vi "一体站流程平行样自动启动.vi"(11 "参数":T1) -> ()   [LabVIEW 2016, in "质控单元.lvlib"]
panel:
  out "枚举":enum16{"初始化", "采配水启动", "等待", "配水", "排水", "结束"}(ring)
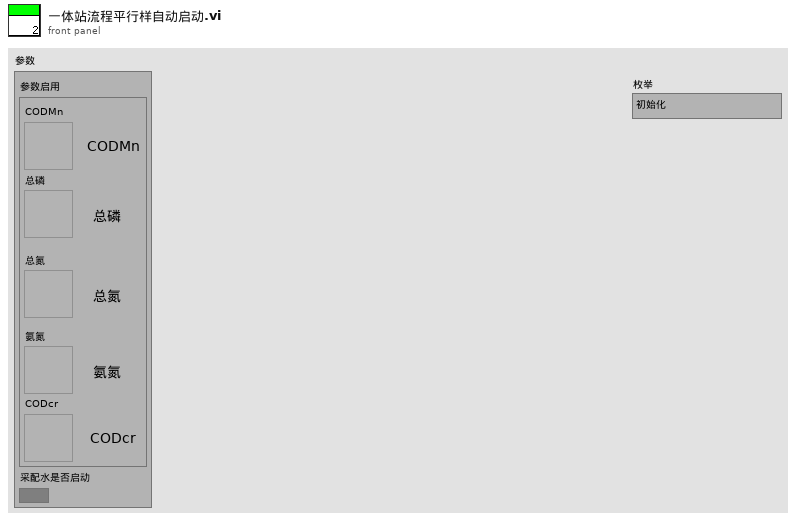
[diagram p1: front panel]
types:
  T1 = cluster{"参数启用":cluster{"CODMn":bool, "总磷":bool, "总氮":bool, "氨氮":bool, "CODcr":bool}, "采配水是否启动":bool}
  T2 = cluster{"命令":string, cluster{"starting address":u16, "holding register value":u16}}
  T3 = typedef "质控单元.lvlib/平行样测试流程.ctl" = enum16{"待机", "第一次水样测试启动", "第一次水样测试中", "第二次水样测试启动", "第二次水样测试中", "存储平行样测试数据", "结束"}
  T4 = cluster{"站号":u16, "量程切换":enum32{"H", "L", "AUTO"}, "控制命令":enum16{"启动测量", "标样核查", "零点核查", "跨度核查", "空白测试", "平行样测试", "加标回收", "空白校准", "标样校准", "初始化（清洗）", "停止测试", "仪器重启", "校时", "模式设置", "测量间隔设置"}, "模式设置":enum16{"待机", "连续模式", "周期模式", "定点模式", "受控模式", "手动模式"}, "测量间隔":u16}
  T5 = cluster{"时间标识":timestamp, "设备":string, "日志信息":string}
  T6 = enum16{"空闲", "水样测试", "标样核查", "零点核查", "跨度核查", "空白测试", "平行样测试", "加标回收", "空白校准", "标样校准", "初始化（清洗）"}
  T7 = cluster{"测量模式":enum16{"水样测量", "标样核查", "零点核查", "跨度核查", "空白测试", "加标回收", "平行样", "校零", "校标"}}
  T8 = cluster{"时间标识":timestamp, "设备":string, "日志信息":string, "流程参数":string}
  T9 = cluster{"R0":i16, "R1":i16, "R2":i16, "R3":i16, "R4":i16, "R5":i16, "R6":i16, "R7":i16, "R8":i16, "R9":i16, "R10":i16, "R11":i16, "R12":i16, "R13":i16, "R14":i16, "R15":i16, "R16":i16, "R17":i16, "R18":i16, "R19":i16, "R20":i16, "R21":i16, "R22":i16, "R23":i16, "R24":i16, "R25":i16, "R26":i16, "R27":i16, "R28":i16, "R29":i16, "R30":i16, "R31":i16, "R32":i16, "R33":i16, "R34":i16, "R35":i16, "R36":i16, "R37":i16, "R38":i16, "R39":i16, "R40":i16, "R41":i16, "R42":i16, "R43":i16, "R44":i16, "R45":i16, "R46":i16, "R47":i16, "R48":i16, "R49":i16, "R50":i16, "R51":i16, "R52":i16, "R53":i16, "R54":i16, "R55":i16, "R56":i16}
  T10 = cluster{"系统时间":timestamp, "工作状态":enum16{"空闲", "水样测试", "标样核查", "零点核查", "跨度核查", "空白测试", "平行样测试", "加标回收", "空白校准", "标样校准", "初始化（清洗）"}, "测量模式":enum16{"待机", "连续模式", "周期模式", "定点模式", "受控模式", "手动模式"}, "告警代码":enum16{"无告警", "缺试剂告警", "缺水样告警", "缺蒸馏水告警", "缺标液告警", "仪表漏液告警", "标定异常告警", "超量程告警", "加热异常", "低试剂预警", "超上限告警", "超下限告警", "仪表内部其他异常", "滴定异常告警", "电极异常告警", "量程切换告警", "参数设置告警", "PH电极电位异常", "电导率电极异常", "浊度光度异常", "溶解氧电极异常", "溶解氧光强异常", "温度异常告警", "PH异常告警", "溶解氧异常告警", "电导率异常告警", "浊度异常告警", "叶绿素异常告警", "藻密度异常告警", "蓝绿藻异常告警", "ORP异常告警", "氨氮异常告警", "清洁刷异常告警", "SD卡异常告警", "蓝牙异常告警", "Wifi异常告警", "流程异常告警"}, "故障代码":enum16{"无故障", "电机故障", "温度故障", "通讯故障", "滴定故障"}, "日志代码":u16, "软件版本":u16, "F0":sgl, "F1":sgl, "F2":sgl, "F3":sgl, "T":sgl, "H":sgl, "id":u16, "flowid":u16, "量程":u16, "总磷控温温度1":sgl, "营养盐控温温度2":sgl, "ADC":sgl}
  T11 = cluster{"因子编码":u32, "单位":u16, "标样参考值":sgl, "水样数据时间":timestamp, "水样实测值":sgl, "水样数据标识":string, "标样数据时间":timestamp, "标样实测值":sgl, "标样数据标识":string, "空白数据时间":timestamp, "空白实测值":sgl, "空白数据标识":string, "零点核查数据时间":timestamp, "零点核查实测值":sgl, "零点核查数据标识":string, "跨度核查数据时间":timestamp, "跨度核查实测值":sgl, "跨度核查数据标识":string, "加标回收数据时间":timestamp, "加标回收实测值":sgl, "加标回收数据标识":string, "平行样数据时间":timestamp, "平行样实测值":sgl, "平行样数据标识":string}
  T12 = cluster{"时间标识":timestamp, "参数":string, "第一次水样浓度值":sgl, "第二次水样测试时间":timestamp, "第二次水样浓度值":sgl}
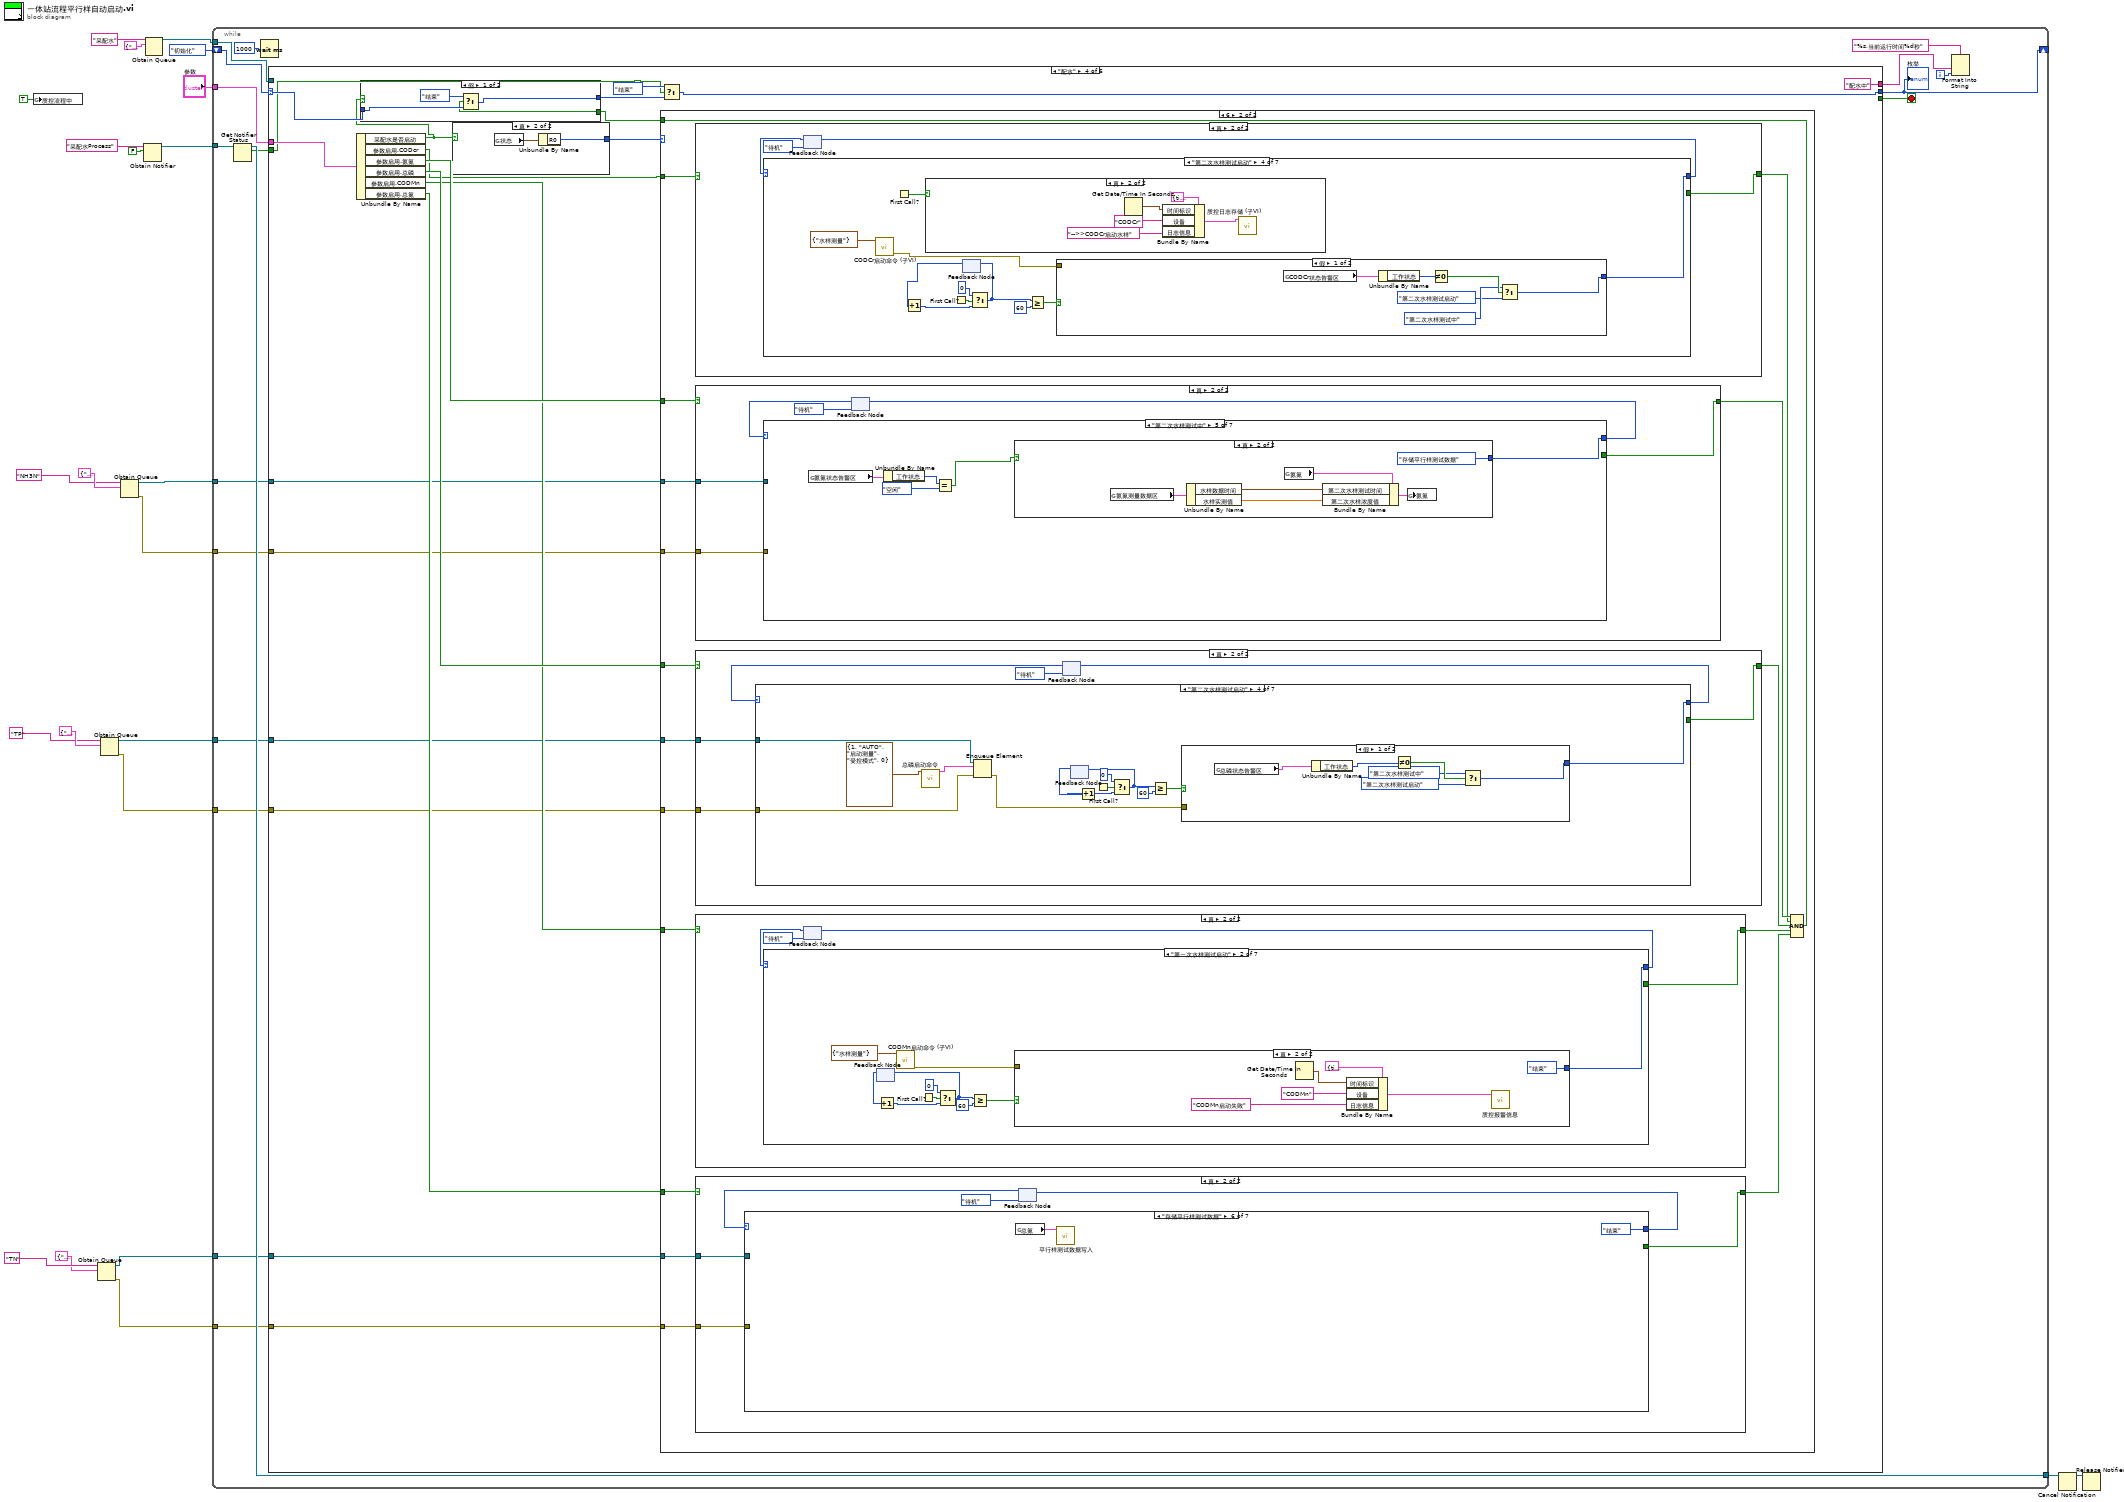
[diagram p0: block diagram]
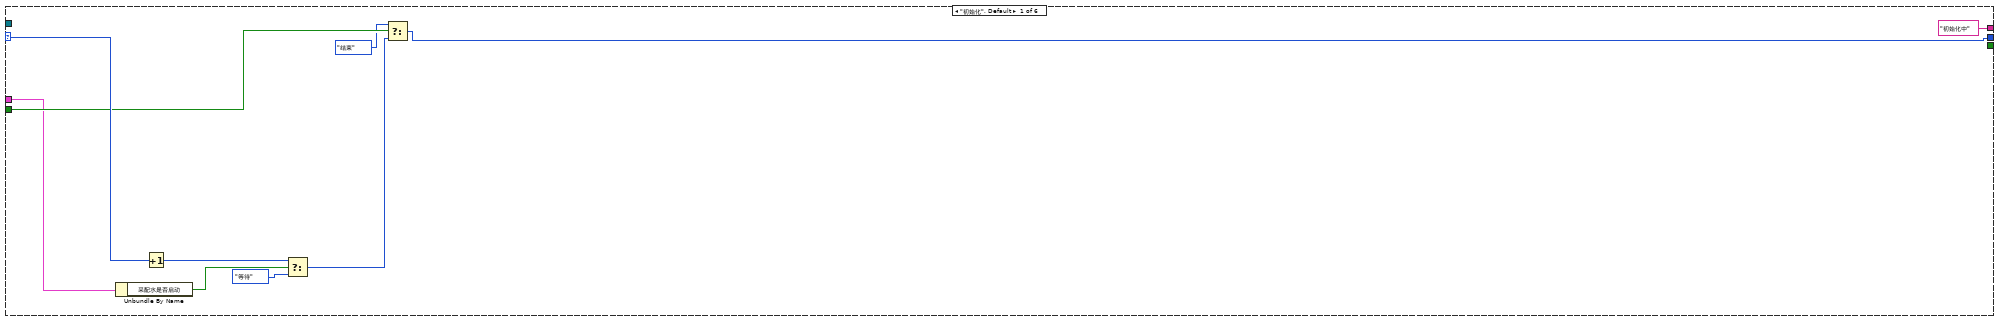
[diagram p2: hidden frame]
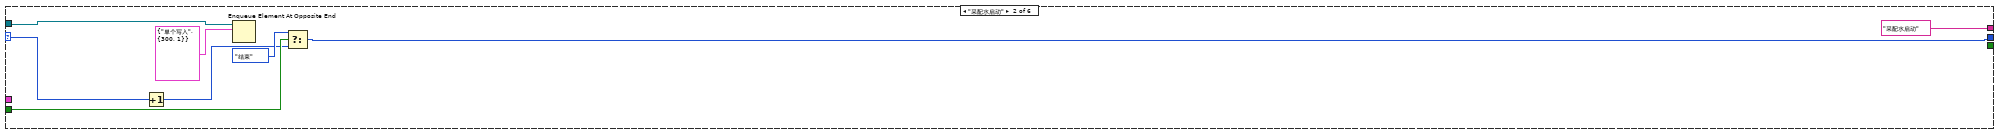
[diagram p3: hidden frame]
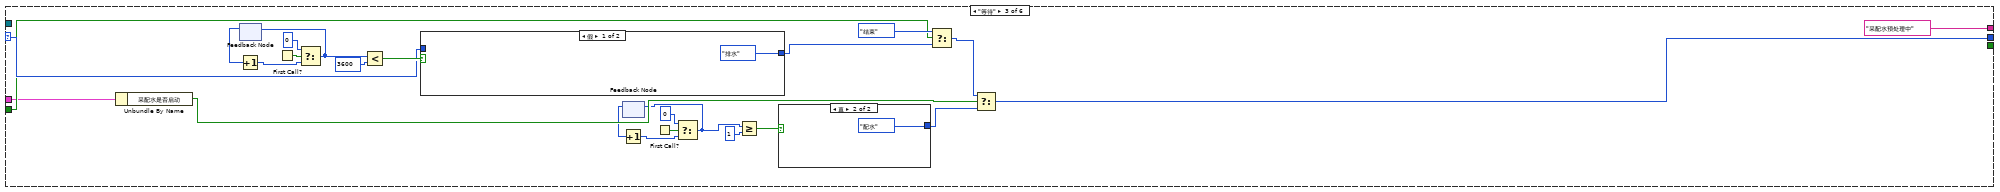
[diagram p4: hidden frame]
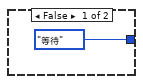
[diagram p5: hidden frame]
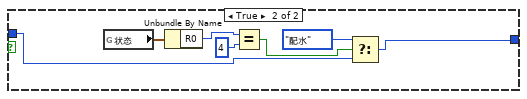
[diagram p6: hidden frame]
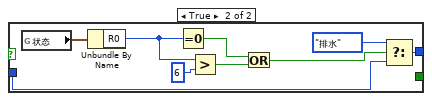
[diagram p7: hidden frame]
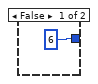
[diagram p8: hidden frame]
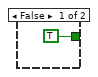
[diagram p10: hidden frame]
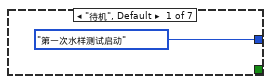
[diagram p11: hidden frame]
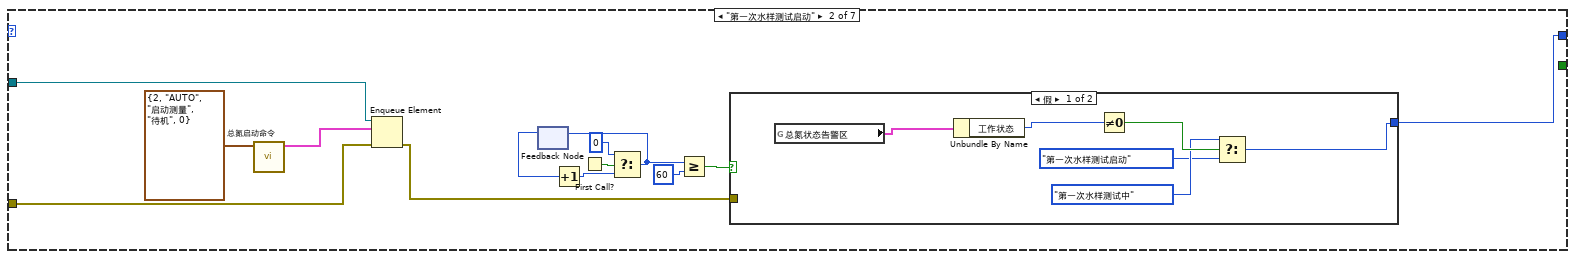
[diagram p12: hidden frame]
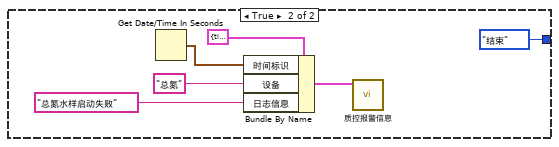
[diagram p13: hidden frame]
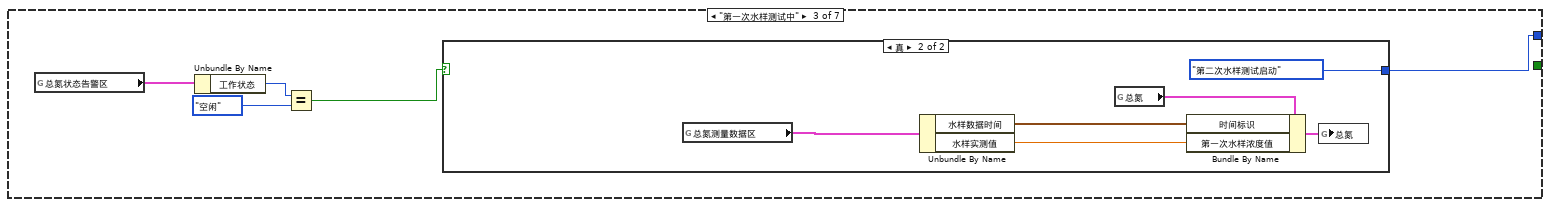
[diagram p14: hidden frame]
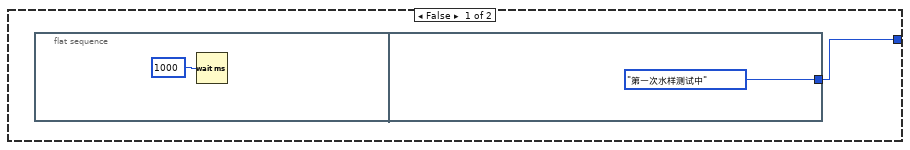
[diagram p15: hidden frame]
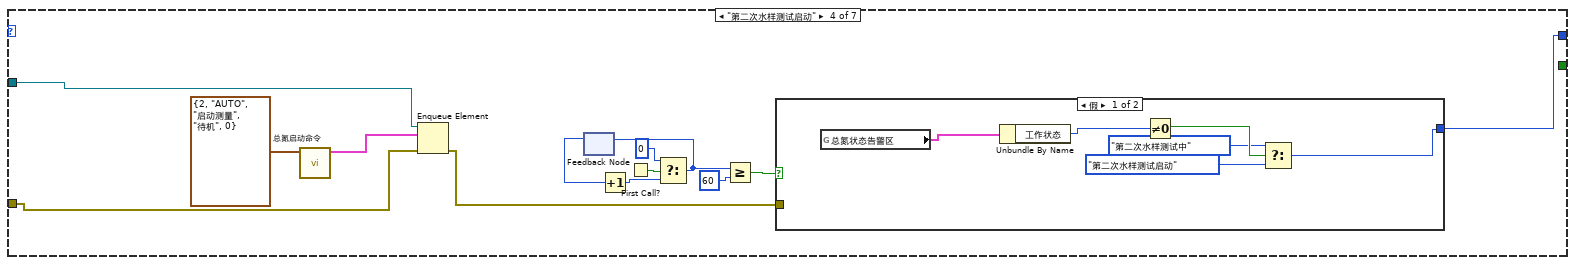
[diagram p16: hidden frame]
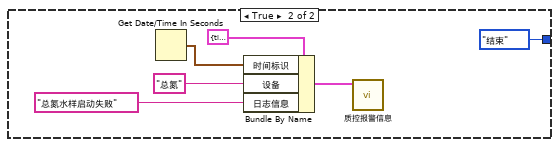
[diagram p17: hidden frame]
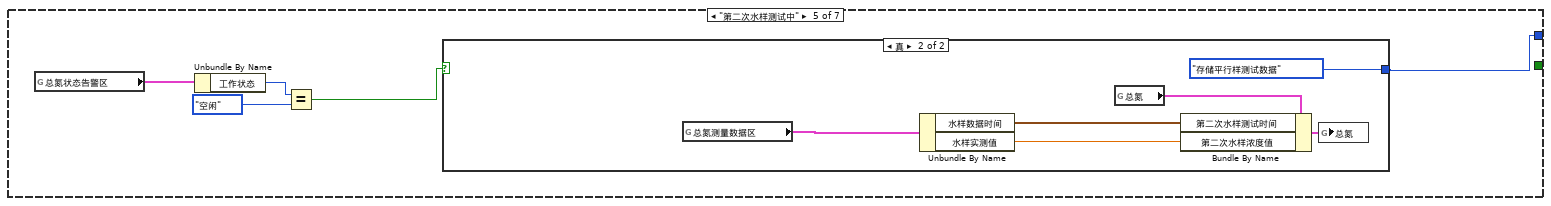
[diagram p18: hidden frame]
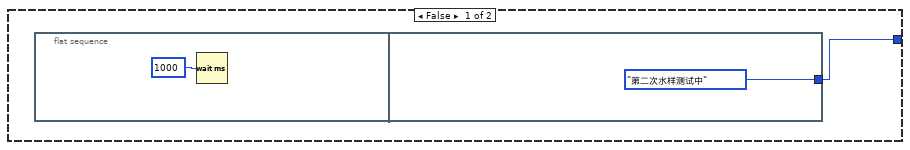
[diagram p19: hidden frame]
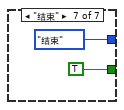
[diagram p20: hidden frame]
diagram:
  n1 = global write "质控测完标志全局 1.vi" "质控流程中"(TRUE ("质控流程中")) -> ()
  n2 = Obtain Queue(name (unnamed)="TN" ("名称（未命名）"), element data type=cluster{"命令":string, "data":variant} {"命令"="", "data"=variant}) -> (queue out=w3:refnum<queue>, error out=w2:errorcluster)  [unwired: 3 in, 1 out]
  n3 = Obtain Queue(name (unnamed)="TP" ("名称（未命名）"), element data type=cluster{"命令":string, "data":variant} {"命令"="", "data"=variant}) -> (queue out=w5:refnum<queue>, error out=w4:errorcluster)  [unwired: 3 in, 1 out]
  n4 = Obtain Queue(name (unnamed)="NH3N" ("名称（未命名）"), element data type=cluster{"命令":string, "data":variant} {"命令"="", "data"=variant}) -> (queue out=w7:refnum<queue>, error out=w6:errorcluster)  [unwired: 3 in, 1 out]
  n5 = Obtain Notifier(name (unnamed)="采配水Process" ("名称（未命名）"), notification data type=FALSE) -> (notifier out=w16:refnum<notifier>)  [unwired: 2 in, 2 out]
  n6 = Obtain Queue(name (unnamed)="采配水" ("名称（未命名）"), element data type=cluster{"命令":string, "数据":variant} {"命令"="", "数据"=variant}) -> (queue out=w21:refnum<queue>)  [unwired: 3 in, 2 out]
  n7 = while {
    tunnel: w21 -> [w41]
    shift-right: [w39] -> _
    shift-left: enum16{"初始化", "采配水启动", "等待", "配水", "排水", "结束"}."初始化" ("枚举") -> [w40]
    tunnel: "参数" -> [w37]
    tunnel: w16 -> [w36]
    tunnel: [w35] -> w15
    tunnel: w7 -> [w30]
    tunnel: w6 -> [w29]
    tunnel: w5 -> [w28]
    tunnel: w4 -> [w27]
    tunnel: w3 -> [w26]
    tunnel: w2 -> [w25]
    i -> [w32]
    stop <- w24 stop-if-true
    n8 = Get Notifier Status(notifier=w36) -> (notifier out=w35:refnum<notifier>, current notification=w31:bool)  [unwired: 1 in, 3 out]
    n9 = Wait (ms)(milliseconds to wait=u32 1000 ("等待时间（毫秒）")) -> ()  [unwired: 1 out]
    n10 = case shown="\"配水\"" w40 {
      selector: w40 -> [w51 w57 w81 w114 w591 w598]
      tunnel: w41 -> [_ w58 _ _ w592 _]
      tunnel: [w48 w52 w60 w111 w586 w597] -> w39
      tunnel: [_ _ _ _ _ TRUE] -> w24
      tunnel: w37 -> [w46 _ w71 w107 _ _]
      tunnel: ["初始化中" ("输入 1") "采配水启动" ("输入 1") "采配水预处理中" ("输入 1") "配水中" ("输入 1") "排水中" ("输入 1") "结束" ("输入 1")] -> w33
      tunnel: w31 -> [w49 w54 w73 w95 w588 _]
      tunnel: w30 -> [_ _ _ w102 _ _]
      tunnel: w29 -> [_ _ _ w101 _ _]
      tunnel: w28 -> [_ _ _ w100 _ _]
      tunnel: w27 -> [_ _ _ w99 _ _]
      tunnel: w26 -> [_ _ _ w98 _ _]
      tunnel: w25 -> [_ _ _ w97 _ _]
      frame "初始化", Default {
        n11 = Unbundle By Name(w46) -> ("采配水是否启动"=w45:bool)
        n12 = Increment(x=w51) -> (x+1=w44:enum16{"初始化", "采配水启动", "等待", "配水", "排水", "结束"})
        n13 = Select(t=w44, s=w45, f=enum16{"初始化", "采配水启动", "等待", "配水", "排水", "结束"}."等待") -> (s? t:f=w43:enum16{"初始化", "采配水启动", "等待", "配水", "排水", "结束"})
        n14 = Select(t=enum16{"初始化", "采配水启动", "等待", "配水", "排水", "结束"}."结束", s=w49, f=w43) -> (s? t:f=w48:enum16{"初始化", "采配水启动", "等待", "配水", "排水", "结束"})
      }
      frame "采配水启动" {
        n15 = Increment(x=w57) -> (x+1=w53:enum16{"初始化", "采配水启动", "等待", "配水", "排水", "结束"})
        n16 = Enqueue Element At Opposite End(queue=w58, element=T2 {"命令"="单个写入", {"starting address"=300, "holding register value"=1}} ("元素")) -> ()  [unwired: 2 in, 3 out]
        n17 = Select(t=enum16{"初始化", "采配水启动", "等待", "配水", "排水", "结束"}."结束", s=w54, f=w53) -> (s? t:f=w52:enum16{"初始化", "采配水启动", "等待", "配水", "排水", "结束"})
      }
      frame "等待" {
        n18 = Unbundle By Name(w71) -> ("采配水是否启动"=w70:bool)
        n19 = feedback #1() -> (w78:i32)  [unwired: 1 in]
        n20 = Increment(x=w78) -> (x+1=w77:i32)
        n21 = First Call?() -> (First Call?: T/F=w79:bool)
        n22 = Select(t=0, s=w79, f=w77) -> (s? t:f=w76:i32)
        n23 = feedback-in #1(w76) -> ()
        n24 = Less?(x=w76, y=3600) -> (x < y?=w82:bool)
        n25 = case shown="假" w82 {
          tunnel: w81 -> [_ w88]
          tunnel: [enum16{"初始化", "采配水启动", "等待", "配水", "排水", "结束"}."排水" ("枚举") w87] -> w72
          frame False {
          }
          frame True {
            n26 = global read "与采配水交互全局.vi" "状态"() -> (w93:T9)
            n27 = Unbundle By Name(w93) -> ("R0"=w92:i16)
            n28 = Equal?(x=w92, y=i16 4) -> (x = y?=w90:bool)
            n29 = Select(t=enum16{"初始化", "采配水启动", "等待", "配水", "排水", "结束"}."配水" ("枚举"), s=w90, f=w88) -> (s? t:f=w87:enum16{"初始化", "采配水启动", "等待", "配水", "排水", "结束"})
          }
        }
        n30 = feedback #2() -> (w66:i32)  [unwired: 1 in]
        n31 = Increment(x=w66) -> (x+1=w67:i32)
        n32 = First Call?() -> (First Call?: T/F=w65:bool)
        n33 = Select(t=0, s=w65, f=w67) -> (s? t:f=w68:i32)
        n34 = feedback-in #2(w68) -> ()
        n35 = Greater Or Equal?(x=w68, y=1) -> (x >= y?=w62:bool)
        n36 = case shown="真" w62 {
          tunnel: [enum16{"初始化", "采配水启动", "等待", "配水", "排水", "结束"}."等待" ("t") enum16{"初始化", "采配水启动", "等待", "配水", "排水", "结束"}."配水" ("t")] -> w61
          frame False {
          }
          frame True {
          }
        }
        n37 = Select(t=enum16{"初始化", "采配水启动", "等待", "配水", "排水", "结束"}."结束", s=w73, f=w72) -> (s? t:f=w69:enum16{"初始化", "采配水启动", "等待", "配水", "排水", "结束"})
        n38 = Select(t=w69, s=w70, f=w61) -> (s? t:f=w60:enum16{"初始化", "采配水启动", "等待", "配水", "排水", "结束"})
      }
      frame "配水" {
        n39 = Unbundle By Name(w107) -> ("采配水是否启动"=w96:bool, "参数启用.CODcr"=w106:bool, "参数启用.氨氮"=w110:bool, "参数启用.总磷"=w109:bool, "参数启用.CODMn"=w108:bool, "参数启用.总氮"=w105:bool)
        n40 = case shown="真" w96 {
          tunnel: [i16 6 ("R0") w129] -> w104
          frame False {
          }
          frame True {
            n41 = global read "与采配水交互全局.vi" "状态"() -> (w130:T9)
            n42 = Unbundle By Name(w130) -> ("R0"=w129:i16)
          }
        }
        n43 = case shown="6" w104 {
          tunnel: w110 -> [_ w147]
          tunnel: w109 -> [_ w146]
          tunnel: w108 -> [_ w143]
          tunnel: w106 -> [_ w142]
          tunnel: w105 -> [_ w139]
          tunnel: w102 -> [_ w137]
          tunnel: w101 -> [_ w136]
          tunnel: w100 -> [_ w135]
          tunnel: w99 -> [_ w134]
          tunnel: w98 -> [_ w133]
          tunnel: w97 -> [_ w132]
          tunnel: [_ w131] -> w94
          frame 0, Default {
          }
          frame 6 {
            n44 = case shown="真" w142 {
              tunnel: [TRUE w314] -> w141
              frame False {
              }
              frame True {
                n45 = feedback #3(平行样测试流程."待机") -> (w316:T3)
                n46 = case shown="\"第二次水样测试启动\"" w316 {
                  tunnel: [平行样测试流程."第一次水样测试启动" w328 w350 w370 w392 平行样测试流程."结束" 平行样测试流程."结束"] -> w315
                  tunnel: [_ _ _ _ _ _ TRUE] -> w314
                  frame "待机", Default {
                  }
                  frame "第一次水样测试启动" {
                    n47 = call "CODCr启动命令 (子VI).vi"("启动测量模式"=T7 {"测量模式"=enum."水样测量"}) -> ("错误输出"=w318:errorcluster)  [unwired: 10 in]
                    n48 = First Call?() -> (First Call?: T/F=w320:bool)
                    n49 = case shown="真" w320 {
                      frame False {
                      }
                      frame True {
                        n50 = Get Date/Time In Seconds() -> (seconds since 1Jan1904=w331:timestamp)
                        n51 = Bundle By Name(cluster=T8 {"时间标识"=timestamp(0 s since 1904-01-01), "设备"="", "日志信息"="", "流程参数"=""} ("data in"), "时间标识"=w331, "设备"="CODCr", "日志信息"="-->>CODCr启动水样") -> (w332:T8)
                        n52 = call "质控日志存储 (子VI).vi"("data in"=w332) -> ()  [unwired: 11 in]
                      }
                    }
                    n53 = feedback #4() -> (w324:i32)  [unwired: 1 in]
                    n54 = Increment(x=w324) -> (x+1=w325:i32)
                    n55 = First Call?() -> (First Call?: T/F=w323:bool)
                    n56 = Select(t=0, s=w323, f=w325) -> (s? t:f=w326:i32)
                    n57 = feedback-in #4(w326) -> ()
                    n58 = Greater Or Equal?(x=w326, y=60) -> (x >= y?=w321:bool)
                    n59 = case shown="假" w321 {
                      tunnel: [w338 平行样测试流程."结束"] -> w328
                      tunnel: w318 -> [_ _]
                      frame False {
                        n60 = global read "与CODCr交互全局.vi" "CODCr状态告警区"() -> (w335:T10)
                        n61 = Unbundle By Name(w335) -> ("工作状态"=w334:T6)
                        n62 = Not Equal To 0?(x=w334) -> (x != 0?=w339:bool)
                        n63 = Select(t=平行样测试流程."第一次水样测试中", s=w339, f=平行样测试流程."第一次水样测试启动") -> (s? t:f=w338:T3)
                      }
                      frame True {
                        n64 = Get Date/Time In Seconds() -> (seconds since 1Jan1904=w342:timestamp)
                        n65 = Bundle By Name(cluster=T5 {"时间标识"=timestamp(0 s since 1904-01-01), "设备"="", "日志信息"=""} ("data in"), "时间标识"=w342, "设备"="CODCr", "日志信息"="CODCr水样启动失败") -> (w340:T5)
                        n66 = call "质控报警信息.vi"("data in"=w340) -> ()  [unwired: 11 in]
                      }
                    }
                  }
                  frame "第一次水样测试中" {
                    n67 = global read "与CODCr交互全局.vi" "CODCr状态告警区"() -> (w349:T10)
                    n68 = Unbundle By Name(w349) -> ("工作状态"=w346:T6)
                    n69 = Equal?(x=w346, y=T6."空闲" ("工作状态")) -> (x = y?=w348:bool)
                    n70 = case shown="真" w348 {
                      tunnel: [w351 平行样测试流程."第二次水样测试启动"] -> w350
                      frame False {
                        n71 = flat-sequence {
                          tunnel: [平行样测试流程."第一次水样测试中"] -> w351
                          frame #0 {
                            n72 = Wait (ms)(milliseconds to wait=u32 1000 ("等待时间（毫秒）")) -> ()  [unwired: 1 out]
                          }
                          frame #1 {
                          }
                        }
                      }
                      frame True {
                        n73 = global read "与CODCr交互全局.vi" "CODCr测量数据区"() -> (w356:T11)
                        n74 = Unbundle By Name(w356) -> ("水样数据时间"=w355:timestamp, "水样实测值"=w354:sgl)
                        n75 = global read "平行样测试全局变量.vi" "CODcr"() -> (w358:T12)
                        n76 = Bundle By Name(cluster=w358, "时间标识"=w355, "第一次水样浓度值"=w354) -> (w357:T12)
                        n77 = global write "平行样测试全局变量.vi" "CODcr"(w357) -> ()
                      }
                    }
                  }
                  frame "第二次水样测试启动" {
                    n78 = call "CODCr启动命令 (子VI).vi"("启动测量模式"=T7 {"测量模式"=enum."水样测量"}) -> ("错误输出"=w360:errorcluster)  [unwired: 10 in]
                    n79 = First Call?() -> (First Call?: T/F=w362:bool)
                    n80 = case shown="真" w362 {
                      frame False {
                      }
                      frame True {
                        n81 = Get Date/Time In Seconds() -> (seconds since 1Jan1904=w373:timestamp)
                        n82 = Bundle By Name(cluster=T8 {"时间标识"=timestamp(0 s since 1904-01-01), "设备"="", "日志信息"="", "流程参数"=""} ("data in"), "时间标识"=w373, "设备"="CODCr", "日志信息"="-->>CODCr启动水样") -> (w374:T8)
                        n83 = call "质控日志存储 (子VI).vi"("data in"=w374) -> ()  [unwired: 11 in]
                      }
                    }
                    n84 = First Call?() -> (First Call?: T/F=w365:bool)
                    n85 = feedback #5() -> (w366:i32)  [unwired: 1 in]
                    n86 = Increment(x=w366) -> (x+1=w367:i32)
                    n87 = Select(t=0, s=w365, f=w367) -> (s? t:f=w368:i32)
                    n88 = feedback-in #5(w368) -> ()
                    n89 = Greater Or Equal?(x=w368, y=60) -> (x >= y?=w363:bool)
                    n90 = case shown="假" w363 {
                      tunnel: [w380 平行样测试流程."结束"] -> w370
                      tunnel: w360 -> [_ _]
                      frame False {
                        n91 = global read "与CODCr交互全局.vi" "CODCr状态告警区"() -> (w377:T10)
                        n92 = Unbundle By Name(w377) -> ("工作状态"=w376:T6)
                        n93 = Not Equal To 0?(x=w376) -> (x != 0?=w381:bool)
                        n94 = Select(t=平行样测试流程."第二次水样测试中", s=w381, f=平行样测试流程."第二次水样测试启动") -> (s? t:f=w380:T3)
                      }
                      frame True {
                        n95 = Get Date/Time In Seconds() -> (seconds since 1Jan1904=w384:timestamp)
                        n96 = Bundle By Name(cluster=T5 {"时间标识"=timestamp(0 s since 1904-01-01), "设备"="", "日志信息"=""} ("data in"), "时间标识"=w384, "设备"="CODCr", "日志信息"="CODCr启动失败") -> (w382:T5)
                        n97 = call "质控报警信息.vi"("data in"=w382) -> ()  [unwired: 11 in]
                      }
                    }
                  }
                  frame "第二次水样测试中" {
                    n98 = global read "与CODCr交互全局.vi" "CODCr状态告警区"() -> (w391:T10)
                    n99 = Unbundle By Name(w391) -> ("工作状态"=w388:T6)
                    n100 = Equal?(x=w388, y=T6."空闲" ("工作状态")) -> (x = y?=w390:bool)
                    n101 = case shown="假" w390 {
                      tunnel: [w393 平行样测试流程."存储平行样测试数据"] -> w392
                      frame False {
                        n102 = flat-sequence {
                          tunnel: [平行样测试流程."第二次水样测试中"] -> w393
                          frame #0 {
                            n103 = Wait (ms)(milliseconds to wait=u32 1000 ("等待时间（毫秒）")) -> ()  [unwired: 1 out]
                          }
                          frame #1 {
                          }
                        }
                      }
                      frame True {
                        n104 = global read "与CODCr交互全局.vi" "CODCr测量数据区"() -> (w398:T11)
                        n105 = Unbundle By Name(w398) -> ("水样数据时间"=w397:timestamp, "水样实测值"=w396:sgl)
                        n106 = global read "平行样测试全局变量.vi" "CODcr"() -> (w400:T12)
                        n107 = Bundle By Name(cluster=w400, "第二次水样测试时间"=w397, "第二次水样浓度值"=w396) -> (w399:T12)
                        n108 = global write "平行样测试全局变量.vi" "CODcr"(w399) -> ()
                      }
                    }
                  }
                  frame "存储平行样测试数据" {
                    n109 = global read "平行样测试全局变量.vi" "CODcr"() -> (w402:T12)
                    n110 = call "平行样测试数据写入.vi"("data"=w402) -> ()  [unwired: 10 in, 1 out]
                  }
                  frame "结束" {
                    n111 = First Call?() -> (First Call?: T/F=w405:bool)
                    n112 = case shown="真" w405 {
                      frame False {
                      }
                      frame True {
                        (unwired) "-->>CODCr停止" ("日志信息")
                        (unwired) "CODCr" ("设备")
                        n113 = call "质控日志存储 (子VI).vi"() -> ()  [unwired: 12 in]
                      }
                    }
                  }
                }
                n114 = feedback-in #3(w315) -> ()
              }
            }
            n115 = case shown="真" w147 {
              tunnel: [TRUE w500] -> w145
              tunnel: w137 -> [_ w499]
              tunnel: w136 -> [_ w498]
              frame False {
              }
              frame True {
                n116 = feedback #6(平行样测试流程."待机") -> (w502:T3)
                n117 = case shown="\"第二次水样测试中\"" w502 {
                  tunnel: [平行样测试流程."第一次水样测试启动" w505 w534 w548 w572 平行样测试流程."结束" 平行样测试流程."结束"] -> w501
                  tunnel: [_ _ _ _ _ _ TRUE] -> w500
                  tunnel: w499 -> [_ w515 _ w545 _ _ _]
                  tunnel: w498 -> [_ w514 _ w544 _ _ _]
                  frame "待机", Default {
                  }
                  frame "第一次水样测试启动" {
                    n118 = call "氨氮启动命令.vi"("参数"=T4 {"站号"=3, "量程切换"=enum."AUTO", "控制命令"=enum."启动测量", "模式设置"=enum."受控模式", "测量间隔"=0}) -> ("启动命令"=w517:cluster{"命令":string, "data":variant})  [unwired: 10 in]
                    n119 = Enqueue Element(queue=w515, element=w517, error in (no error)=w514) -> (error out=w506:errorcluster)  [unwired: 1 in, 2 out]
                    n120 = feedback #7() -> (w510:i32)  [unwired: 1 in]
                    n121 = Increment(x=w510) -> (x+1=w511:i32)
                    n122 = First Call?() -> (First Call?: T/F=w509:bool)
                    n123 = Select(t=0, s=w509, f=w511) -> (s? t:f=w512:i32)
                    n124 = feedback-in #7(w512) -> ()
                    n125 = Greater Or Equal?(x=w512, y=60) -> (x >= y?=w507:bool)
                    n126 = case shown="假" w507 {
                      tunnel: [w522 平行样测试流程."结束"] -> w505
                      tunnel: w506 -> [_ _]
                      frame False {
                        n127 = global read "与氨氮交互全局.vi" "氨氮状态告警区"() -> (w518:T10)
                        n128 = Unbundle By Name(w518) -> ("工作状态"=w519:T6)
                        n129 = Not Equal To 0?(x=w519) -> (x != 0?=w523:bool)
                        n130 = Select(t=平行样测试流程."第一次水样测试中", s=w523, f=平行样测试流程."第一次水样测试启动") -> (s? t:f=w522:T3)
                      }
                      frame True {
                        n131 = Get Date/Time In Seconds() -> (seconds since 1Jan1904=w526:timestamp)
                        n132 = Bundle By Name(cluster=T5 {"时间标识"=timestamp(0 s since 1904-01-01), "设备"="", "日志信息"=""} ("data in"), "时间标识"=w526, "设备"="氨氮", "日志信息"="氨氮水样启动失败") -> (w524:T5)
                        n133 = call "质控报警信息.vi"("data in"=w524) -> ()  [unwired: 11 in]
                      }
                    }
                  }
                  frame "第一次水样测试中" {
                    n134 = global read "与氨氮交互全局.vi" "氨氮状态告警区"() -> (w533:T10)
                    n135 = Unbundle By Name(w533) -> ("工作状态"=w531:T6)
                    n136 = Equal?(x=w531, y=T6."空闲" ("工作状态")) -> (x = y?=w530:bool)
                    n137 = case shown="真" w530 {
                      tunnel: [w535 平行样测试流程."第二次水样测试启动"] -> w534
                      frame False {
                        n138 = flat-sequence {
                          tunnel: [平行样测试流程."第一次水样测试中"] -> w535
                          frame #0 {
                            n139 = Wait (ms)(milliseconds to wait=u32 1000 ("等待时间（毫秒）")) -> ()  [unwired: 1 out]
                          }
                          frame #1 {
                          }
                        }
                      }
                      frame True {
                        n140 = global read "与氨氮交互全局.vi" "氨氮测量数据区"() -> (w540:T11)
                        n141 = Unbundle By Name(w540) -> ("水样数据时间"=w539:timestamp, "水样实测值"=w538:sgl)
                        n142 = global read "平行样测试全局变量.vi" "氨氮"() -> (w542:T12)
                        n143 = Bundle By Name(cluster=w542, "时间标识"=w539, "第一次水样浓度值"=w538) -> (w541:T12)
                        n144 = global write "平行样测试全局变量.vi" "氨氮"(w541) -> ()
                      }
                    }
                  }
                  frame "第二次水样测试启动" {
                    n145 = call "氨氮启动命令.vi"("参数"=T4 {"站号"=3, "量程切换"=enum."AUTO", "控制命令"=enum."启动测量", "模式设置"=enum."受控模式", "测量间隔"=0}) -> ("启动命令"=w547:cluster{"命令":string, "data":variant})  [unwired: 10 in]
                    n146 = Enqueue Element(queue=w545, element=w547, error in (no error)=w544) -> ()  [unwired: 1 in, 3 out]
                    n147 = feedback #8() -> (w552:i32)  [unwired: 1 in]
                    n148 = Increment(x=w552) -> (x+1=w553:i32)
                    n149 = First Call?() -> (First Call?: T/F=w551:bool)
                    n150 = Select(t=0, s=w551, f=w553) -> (s? t:f=w554:i32)
                    n151 = feedback-in #8(w554) -> ()
                    n152 = Greater Or Equal?(x=w554, y=60) -> (x >= y?=w549:bool)
                    n153 = case shown="假" w549 {
                      tunnel: [w558 平行样测试流程."结束"] -> w548
                      frame False {
                        n154 = global read "与氨氮交互全局.vi" "氨氮状态告警区"() -> (w561:T10)
                        n155 = Unbundle By Name(w561) -> ("工作状态"=w557:T6)
                        n156 = Not Equal To 0?(x=w557) -> (x != 0?=w556:bool)
                        n157 = Select(t=平行样测试流程."第二次水样测试中", s=w556, f=平行样测试流程."第二次水样测试启动") -> (s? t:f=w558:T3)
                      }
                      frame True {
                        n158 = Get Date/Time In Seconds() -> (seconds since 1Jan1904=w564:timestamp)
                        n159 = Bundle By Name(cluster=T5 {"时间标识"=timestamp(0 s since 1904-01-01), "设备"="", "日志信息"=""} ("data in"), "时间标识"=w564, "设备"="氨氮", "日志信息"="氨氮水样启动失败") -> (w563:T5)
                        n160 = call "质控报警信息.vi"("data in"=w563) -> ()  [unwired: 11 in]
                      }
                    }
                  }
                  frame "第二次水样测试中" {
                    n161 = global read "与氨氮交互全局.vi" "氨氮状态告警区"() -> (w571:T10)
                    n162 = Unbundle By Name(w571) -> ("工作状态"=w569:T6)
                    n163 = Equal?(x=w569, y=T6."空闲" ("工作状态")) -> (x = y?=w568:bool)
                    n164 = case shown="真" w568 {
                      tunnel: [w573 平行样测试流程."存储平行样测试数据"] -> w572
                      frame False {
                        n165 = flat-sequence {
                          tunnel: [平行样测试流程."第二次水样测试中"] -> w573
                          frame #0 {
                            n166 = Wait (ms)(milliseconds to wait=u32 1000 ("等待时间（毫秒）")) -> ()  [unwired: 1 out]
                          }
                          frame #1 {
                          }
                        }
                      }
                      frame True {
                        n167 = global read "与氨氮交互全局.vi" "氨氮测量数据区"() -> (w578:T11)
                        n168 = Unbundle By Name(w578) -> ("水样数据时间"=w577:timestamp, "水样实测值"=w576:sgl)
                        n169 = global read "平行样测试全局变量.vi" "氨氮"() -> (w580:T12)
                        n170 = Bundle By Name(cluster=w580, "第二次水样测试时间"=w577, "第二次水样浓度值"=w576) -> (w579:T12)
                        n171 = global write "平行样测试全局变量.vi" "氨氮"(w579) -> ()
                      }
                    }
                  }
                  frame "存储平行样测试数据" {
                    n172 = global read "平行样测试全局变量.vi" "氨氮"() -> (w582:T12)
                    n173 = call "平行样测试数据写入.vi"("data"=w582) -> ()  [unwired: 10 in, 1 out]
                  }
                  frame "结束" {
                  }
                }
                n174 = feedback-in #6(w501) -> ()
              }
            }
            n175 = case shown="真" w146 {
              tunnel: [TRUE w411] -> w144
              tunnel: w135 -> [_ w409]
              tunnel: w134 -> [_ w408]
              frame False {
              }
              frame True {
                n176 = feedback #9(平行样测试流程."待机") -> (w413:T3)
                n177 = case shown="\"第二次水样测试启动\"" w413 {
                  tunnel: [平行样测试流程."第一次水样测试启动" w415 w444 w454 w479 平行样测试流程."结束" 平行样测试流程."结束"] -> w412
                  tunnel: [_ _ _ _ _ _ TRUE] -> w411
                  tunnel: w409 -> [_ w427 _ w456 _ _ _]
                  tunnel: w408 -> [_ w426 _ w455 _ _ _]
                  frame "待机", Default {
                  }
                  frame "第一次水样测试启动" {
                    n178 = call "总磷启动命令.vi"("参数"=T4 {"站号"=1, "量程切换"=enum."AUTO", "控制命令"=enum."启动测量", "模式设置"=enum."受控模式", "测量间隔"=0}) -> ("启动命令"=w425:cluster{"命令":string, "data":variant})  [unwired: 10 in]
                    n179 = Enqueue Element(queue=w427, element=w425, error in (no error)=w426) -> (error out=w416:errorcluster)  [unwired: 1 in, 2 out]
                    n180 = feedback #10() -> (w420:i32)  [unwired: 1 in]
                    n181 = Increment(x=w420) -> (x+1=w419:i32)
                    n182 = First Call?() -> (First Call?: T/F=w421:bool)
                    n183 = Select(t=0, s=w421, f=w419) -> (s? t:f=w418:i32)
                    n184 = feedback-in #10(w418) -> ()
                    n185 = Greater Or Equal?(x=w418, y=60) -> (x >= y?=w423:bool)
                    n186 = case shown="假" w423 {
                      tunnel: [w432 平行样测试流程."结束"] -> w415
                      tunnel: w416 -> [_ _]
                      frame False {
                        n187 = global read "与总磷交互全局.vi" "总磷状态告警区"() -> (w428:T10)
                        n188 = Unbundle By Name(w428) -> ("工作状态"=w429:T6)
                        n189 = Not Equal To 0?(x=w429) -> (x != 0?=w433:bool)
                        n190 = Select(t=平行样测试流程."第一次水样测试中", s=w433, f=平行样测试流程."第一次水样测试启动") -> (s? t:f=w432:T3)
                      }
                      frame True {
                        n191 = Get Date/Time In Seconds() -> (seconds since 1Jan1904=w436:timestamp)
                        n192 = Bundle By Name(cluster=T5 {"时间标识"=timestamp(0 s since 1904-01-01), "设备"="", "日志信息"=""} ("data in"), "时间标识"=w436, "设备"="总磷", "日志信息"="总磷水样启动失败") -> (w434:T5)
                        n193 = call "质控报警信息.vi"("data in"=w434) -> ()  [unwired: 11 in]
                      }
                    }
                  }
                  frame "第一次水样测试中" {
                    n194 = global read "与总磷交互全局.vi" "总磷状态告警区"() -> (w440:T10)
                    n195 = Unbundle By Name(w440) -> ("工作状态"=w443:T6)
                    n196 = Equal?(x=w443, y=T6."空闲" ("工作状态")) -> (x = y?=w441:bool)
                    n197 = case shown="真" w441 {
                      tunnel: [w445 平行样测试流程."第二次水样测试启动"] -> w444
                      frame False {
                        n198 = flat-sequence {
                          tunnel: [平行样测试流程."第一次水样测试中"] -> w445
                          frame #0 {
                            n199 = Wait (ms)(milliseconds to wait=u32 1000 ("等待时间（毫秒）")) -> ()  [unwired: 1 out]
                          }
                          frame #1 {
                          }
                        }
                      }
                      frame True {
                        n200 = global read "与总磷交互全局.vi" "总磷测量数据区"() -> (w448:T11)
                        n201 = Unbundle By Name(w448) -> ("水样数据时间"=w451:timestamp, "水样实测值"=w452:sgl)
                        n202 = global read "平行样测试全局变量.vi" "总磷"() -> (w449:T12)
                        n203 = Bundle By Name(cluster=w449, "时间标识"=w451, "第一次水样浓度值"=w452) -> (w450:T12)
                        n204 = global write "平行样测试全局变量.vi" "总磷"(w450) -> ()
                      }
                    }
                  }
                  frame "第二次水样测试启动" {
                    n205 = call "总磷启动命令.vi"("参数"=T4 {"站号"=1, "量程切换"=enum."AUTO", "控制命令"=enum."启动测量", "模式设置"=enum."受控模式", "测量间隔"=0}) -> ("启动命令"=w466:cluster{"命令":string, "data":variant})  [unwired: 10 in]
                    n206 = Enqueue Element(queue=w456, element=w466, error in (no error)=w455) -> (error out=w457:errorcluster)  [unwired: 1 in, 2 out]
                    n207 = feedback #11() -> (w461:i32)  [unwired: 1 in]
                    n208 = Increment(x=w461) -> (x+1=w460:i32)
                    n209 = First Call?() -> (First Call?: T/F=w462:bool)
                    n210 = Select(t=0, s=w462, f=w460) -> (s? t:f=w459:i32)
                    n211 = feedback-in #11(w459) -> ()
                    n212 = Greater Or Equal?(x=w459, y=60) -> (x >= y?=w464:bool)
                    n213 = case shown="假" w464 {
                      tunnel: [w471 平行样测试流程."结束"] -> w454
                      tunnel: w457 -> [_ _]
                      frame False {
                        n214 = global read "与总磷交互全局.vi" "总磷状态告警区"() -> (w467:T10)
                        n215 = Unbundle By Name(w467) -> ("工作状态"=w468:T6)
                        n216 = Not Equal To 0?(x=w468) -> (x != 0?=w472:bool)
                        n217 = Select(t=平行样测试流程."第二次水样测试中", s=w472, f=平行样测试流程."第二次水样测试启动") -> (s? t:f=w471:T3)
                      }
                      frame True {
                        n218 = Get Date/Time In Seconds() -> (seconds since 1Jan1904=w475:timestamp)
                        n219 = Bundle By Name(cluster=T5 {"时间标识"=timestamp(0 s since 1904-01-01), "设备"="", "日志信息"=""} ("data in"), "时间标识"=w475, "设备"="总磷", "日志信息"="总磷水样启动失败") -> (w473:T5)
                        n220 = call "质控报警信息.vi"("data in"=w473) -> ()  [unwired: 11 in]
                      }
                    }
                  }
                  frame "第二次水样测试中" {
                    n221 = global read "与总磷交互全局.vi" "总磷状态告警区"() -> (w480:T10)
                    n222 = Unbundle By Name(w480) -> ("工作状态"=w483:T6)
                    n223 = Equal?(x=w483, y=T6."空闲" ("工作状态")) -> (x = y?=w481:bool)
                    n224 = case shown="真" w481 {
                      tunnel: [w484 平行样测试流程."存储平行样测试数据"] -> w479
                      frame False {
                        n225 = flat-sequence {
                          tunnel: [平行样测试流程."第二次水样测试中"] -> w484
                          frame #0 {
                            n226 = Wait (ms)(milliseconds to wait=u32 1000 ("等待时间（毫秒）")) -> ()  [unwired: 1 out]
                          }
                          frame #1 {
                          }
                        }
                      }
                      frame True {
                        n227 = global read "与总磷交互全局.vi" "总磷测量数据区"() -> (w487:T11)
                        n228 = Unbundle By Name(w487) -> ("水样数据时间"=w490:timestamp, "水样实测值"=w491:sgl)
                        n229 = global read "平行样测试全局变量.vi" "总磷"() -> (w488:T12)
                        n230 = Bundle By Name(cluster=w488, "第二次水样测试时间"=w490, "第二次水样浓度值"=w491) -> (w489:T12)
                        n231 = global write "平行样测试全局变量.vi" "总磷"(w489) -> ()
                      }
                    }
                  }
                  frame "存储平行样测试数据" {
                    n232 = global read "平行样测试全局变量.vi" "总磷"() -> (w493:T12)
                    n233 = call "平行样测试数据写入.vi"("data"=w493) -> ()  [unwired: 10 in, 1 out]
                  }
                  frame "结束" {
                  }
                }
                n234 = feedback-in #9(w412) -> ()
              }
            }
            n235 = case shown="真" w143 {
              tunnel: [TRUE w240] -> w140
              frame False {
              }
              frame True {
                n236 = feedback #12(平行样测试流程."待机") -> (w242:T3)
                n237 = case shown="\"第一次水样测试启动\"" w242 {
                  tunnel: [平行样测试流程."第一次水样测试启动" w253 w267 w285 w299 平行样测试流程."结束" 平行样测试流程."结束"] -> w241
                  tunnel: [_ _ _ _ _ _ TRUE] -> w240
                  frame "待机", Default {
                  }
                  frame "第一次水样测试启动" {
                    n238 = feedback #13() -> (w249:i32)  [unwired: 1 in]
                    n239 = Increment(x=w249) -> (x+1=w250:i32)
                    n240 = call "CODMn启动命令 (子VI).vi"("启动测量模式"=T7 {"测量模式"=enum."水样测量"}) -> ("错误输出"=w244:errorcluster)  [unwired: 10 in]
                    n241 = First Call?() -> (First Call?: T/F=w248:bool)
                    n242 = Select(t=0, s=w248, f=w250) -> (s? t:f=w251:i32)
                    n243 = feedback-in #13(w251) -> ()
                    n244 = Greater Or Equal?(x=w251, y=60) -> (x >= y?=w246:bool)
                    n245 = case shown="真" w246 {
                      tunnel: [w257 平行样测试流程."结束"] -> w253
                      tunnel: w244 -> [_ _]
                      frame False {
                        n246 = global read "与CODMn交互全局.vi" "多列列表框"() -> (w256:i32)
                        n247 = Not Equal To 0?(x=w256) -> (x != 0?=w258:bool)
                        n248 = Select(t=平行样测试流程."第一次水样测试中", s=w258, f=平行样测试流程."第一次水样测试启动") -> (s? t:f=w257:T3)
                      }
                      frame True {
                        n249 = Get Date/Time In Seconds() -> (seconds since 1Jan1904=w261:timestamp)
                        n250 = Bundle By Name(cluster=T5 {"时间标识"=timestamp(0 s since 1904-01-01), "设备"="", "日志信息"=""} ("data in"), "时间标识"=w261, "设备"="CODMn", "日志信息"="CODMn启动失败") -> (w259:T5)
                        n251 = call "质控报警信息.vi"("data in"=w259) -> ()  [unwired: 11 in]
                      }
                    }
                  }
                  frame "第一次水样测试中" {
                    n252 = global read "与CODMn交互全局.vi" "多列列表框"() -> (w266:i32)
                    n253 = Equal To 0?(x=w266) -> (x = 0?=w265:bool)
                    n254 = case shown="假" w265 {
                      tunnel: [w268 平行样测试流程."第二次水样测试启动"] -> w267
                      frame False {
                        n255 = flat-sequence {
                          tunnel: [平行样测试流程."第一次水样测试中"] -> w268
                          frame #0 {
                            n256 = Wait (ms)(milliseconds to wait=u32 1000 ("等待时间（毫秒）")) -> ()  [unwired: 1 out]
                          }
                          frame #1 {
                          }
                        }
                      }
                      frame True {
                        n257 = global read "与CODMn交互全局.vi" "COD浓度（mg/L)"() -> (w271:dbl)
                        n258 = global read "与CODMn交互全局.vi" "水样启动时间"() -> (w272:timestamp)
                        n259 = global read "平行样测试全局变量.vi" "CODMn"() -> (w274:T12)
                        n260 = Bundle By Name(cluster=w274, "时间标识"=w272, "第一次水样浓度值"=w271) -> (w273:T12)
                        n261 = global write "平行样测试全局变量.vi" "CODMn"(w273) -> ()
                      }
                    }
                  }
                  frame "第二次水样测试启动" {
                    n262 = feedback #14() -> (w281:i32)  [unwired: 1 in]
                    n263 = Increment(x=w281) -> (x+1=w282:i32)
                    n264 = First Call?() -> (First Call?: T/F=w280:bool)
                    n265 = call "CODMn启动命令 (子VI).vi"("启动测量模式"=T7 {"测量模式"=enum."水样测量"}) -> ("错误输出"=w276:errorcluster)  [unwired: 10 in]
                    n266 = Select(t=0, s=w280, f=w282) -> (s? t:f=w283:i32)
                    n267 = feedback-in #14(w283) -> ()
                    n268 = Greater Or Equal?(x=w283, y=60) -> (x >= y?=w278:bool)
                    n269 = case shown="真" w278 {
                      tunnel: [w289 平行样测试流程."结束"] -> w285
                      tunnel: w276 -> [_ _]
                      frame False {
                        n270 = global read "与CODMn交互全局.vi" "多列列表框"() -> (w288:i32)
                        n271 = Not Equal To 0?(x=w288) -> (x != 0?=w290:bool)
                        n272 = Select(t=平行样测试流程."第二次水样测试中", s=w290, f=平行样测试流程."第二次水样测试启动") -> (s? t:f=w289:T3)
                      }
                      frame True {
                        n273 = Get Date/Time In Seconds() -> (seconds since 1Jan1904=w293:timestamp)
                        n274 = Bundle By Name(cluster=T5 {"时间标识"=timestamp(0 s since 1904-01-01), "设备"="", "日志信息"=""} ("data in"), "时间标识"=w293, "设备"="CODMn", "日志信息"="CODMn启动失败") -> (w291:T5)
                        n275 = call "质控报警信息.vi"("data in"=w291) -> ()  [unwired: 11 in]
                      }
                    }
                  }
                  frame "第二次水样测试中" {
                    n276 = global read "与CODMn交互全局.vi" "多列列表框"() -> (w298:i32)
                    n277 = Equal To 0?(x=w298) -> (x = 0?=w297:bool)
                    n278 = case shown="真" w297 {
                      tunnel: [w300 平行样测试流程."存储平行样测试数据"] -> w299
                      frame False {
                        n279 = flat-sequence {
                          tunnel: [平行样测试流程."第二次水样测试中"] -> w300
                          frame #0 {
                            n280 = Wait (ms)(milliseconds to wait=u32 1000 ("等待时间（毫秒）")) -> ()  [unwired: 1 out]
                          }
                          frame #1 {
                          }
                        }
                      }
                      frame True {
                        n281 = global read "与CODMn交互全局.vi" "COD浓度（mg/L)"() -> (w303:dbl)
                        n282 = global read "与CODMn交互全局.vi" "水样启动时间"() -> (w304:timestamp)
                        n283 = global read "平行样测试全局变量.vi" "CODMn"() -> (w306:T12)
                        n284 = Bundle By Name(cluster=w306, "时间标识"=w304, "第一次水样浓度值"=w303) -> (w305:T12)
                        n285 = global write "平行样测试全局变量.vi" "CODMn"(w305) -> ()
                      }
                    }
                  }
                  frame "存储平行样测试数据" {
                    n286 = global read "平行样测试全局变量.vi" "CODMn"() -> (w308:T12)
                    n287 = call "平行样测试数据写入.vi"("data"=w308) -> ()  [unwired: 10 in, 1 out]
                  }
                  frame "结束" {
                  }
                }
                n288 = feedback-in #12(w241) -> ()
              }
            }
            n289 = case shown="真" w139 {
              tunnel: [TRUE w152] -> w138
              tunnel: w133 -> [_ w150]
              tunnel: w132 -> [_ w149]
              frame False {
              }
              frame True {
                n290 = feedback #15(平行样测试流程."待机") -> (w154:T3)
                n291 = case shown="\"存储平行样测试数据\"" w154 {
                  tunnel: [平行样测试流程."第一次水样测试启动" w156 w182 w195 w220 平行样测试流程."结束" 平行样测试流程."结束"] -> w153
                  tunnel: [_ _ _ _ _ _ TRUE] -> w152
                  tunnel: w150 -> [_ w160 _ w197 _ _ _]
                  tunnel: w149 -> [_ w159 _ w196 _ _ _]
                  frame "待机", Default {
                  }
                  frame "第一次水样测试启动" {
                    n292 = call "总氮启动命令.vi"("参数"=T4 {"站号"=2, "量程切换"=enum."AUTO", "控制命令"=enum."启动测量", "模式设置"=enum."待机", "测量间隔"=0}) -> ("启动命令"=w158:cluster{"命令":string, "data":variant})  [unwired: 10 in]
                    n293 = Enqueue Element(queue=w160, element=w158, error in (no error)=w159) -> (error out=w161:errorcluster)  [unwired: 1 in, 2 out]
                    n294 = feedback #16() -> (w165:i32)  [unwired: 1 in]
                    n295 = Increment(x=w165) -> (x+1=w164:i32)
                    n296 = First Call?() -> (First Call?: T/F=w166:bool)
                    n297 = Select(t=0, s=w166, f=w164) -> (s? t:f=w163:i32)
                    n298 = feedback-in #16(w163) -> ()
                    n299 = Greater Or Equal?(x=w163, y=60) -> (x >= y?=w168:bool)
                    n300 = case shown="假" w168 {
                      tunnel: [w173 平行样测试流程."结束"] -> w156
                      tunnel: w161 -> [_ _]
                      frame False {
                        n301 = global read "与总氮交互全局.vi" "总氮状态告警区"() -> (w169:T10)
                        n302 = Unbundle By Name(w169) -> ("工作状态"=w170:T6)
                        n303 = Not Equal To 0?(x=w170) -> (x != 0?=w174:bool)
                        n304 = Select(t=平行样测试流程."第一次水样测试中", s=w174, f=平行样测试流程."第一次水样测试启动") -> (s? t:f=w173:T3)
                      }
                      frame True {
                        n305 = Get Date/Time In Seconds() -> (seconds since 1Jan1904=w177:timestamp)
                        n306 = Bundle By Name(cluster=T5 {"时间标识"=timestamp(0 s since 1904-01-01), "设备"="", "日志信息"=""} ("data in"), "时间标识"=w177, "设备"="总氮", "日志信息"="总氮水样启动失败") -> (w175:T5)
                        n307 = call "质控报警信息.vi"("data in"=w175) -> ()  [unwired: 11 in]
                      }
                    }
                  }
                  frame "第一次水样测试中" {
                    n308 = global read "与总氮交互全局.vi" "总氮状态告警区"() -> (w181:T10)
                    n309 = Unbundle By Name(w181) -> ("工作状态"=w185:T6)
                    n310 = Equal?(x=w185, y=T6."空闲" ("工作状态")) -> (x = y?=w183:bool)
                    n311 = case shown="真" w183 {
                      tunnel: [w186 平行样测试流程."第二次水样测试启动"] -> w182
                      frame False {
                        n312 = flat-sequence {
                          tunnel: [平行样测试流程."第一次水样测试中"] -> w186
                          frame #0 {
                            n313 = Wait (ms)(milliseconds to wait=u32 1000 ("等待时间（毫秒）")) -> ()  [unwired: 1 out]
                          }
                          frame #1 {
                          }
                        }
                      }
                      frame True {
                        n314 = global read "与总氮交互全局.vi" "总氮测量数据区"() -> (w189:T11)
                        n315 = Unbundle By Name(w189) -> ("水样数据时间"=w192:timestamp, "水样实测值"=w193:sgl)
                        n316 = global read "平行样测试全局变量.vi" "总氮"() -> (w190:T12)
                        n317 = Bundle By Name(cluster=w190, "时间标识"=w192, "第一次水样浓度值"=w193) -> (w191:T12)
                        n318 = global write "平行样测试全局变量.vi" "总氮"(w191) -> ()
                      }
                    }
                  }
                  frame "第二次水样测试启动" {
                    n319 = call "总氮启动命令.vi"("参数"=T4 {"站号"=2, "量程切换"=enum."AUTO", "控制命令"=enum."启动测量", "模式设置"=enum."待机", "测量间隔"=0}) -> ("启动命令"=w199:cluster{"命令":string, "data":variant})  [unwired: 10 in]
                    n320 = Enqueue Element(queue=w197, element=w199, error in (no error)=w196) -> (error out=w200:errorcluster)  [unwired: 1 in, 2 out]
                    n321 = feedback #17() -> (w204:i32)  [unwired: 1 in]
                    n322 = Increment(x=w204) -> (x+1=w203:i32)
                    n323 = First Call?() -> (First Call?: T/F=w205:bool)
                    n324 = Select(t=0, s=w205, f=w203) -> (s? t:f=w202:i32)
                    n325 = feedback-in #17(w202) -> ()
                    n326 = Greater Or Equal?(x=w202, y=60) -> (x >= y?=w207:bool)
                    n327 = case shown="假" w207 {
                      tunnel: [w212 平行样测试流程."结束"] -> w195
                      tunnel: w200 -> [_ _]
                      frame False {
                        n328 = global read "与总氮交互全局.vi" "总氮状态告警区"() -> (w208:T10)
                        n329 = Unbundle By Name(w208) -> ("工作状态"=w209:T6)
                        n330 = Not Equal To 0?(x=w209) -> (x != 0?=w213:bool)
                        n331 = Select(t=平行样测试流程."第二次水样测试中", s=w213, f=平行样测试流程."第二次水样测试启动") -> (s? t:f=w212:T3)
                      }
                      frame True {
                        n332 = Get Date/Time In Seconds() -> (seconds since 1Jan1904=w216:timestamp)
                        n333 = Bundle By Name(cluster=T5 {"时间标识"=timestamp(0 s since 1904-01-01), "设备"="", "日志信息"=""} ("data in"), "时间标识"=w216, "设备"="总氮", "日志信息"="总氮水样启动失败") -> (w214:T5)
                        n334 = call "质控报警信息.vi"("data in"=w214) -> ()  [unwired: 11 in]
                      }
                    }
                  }
                  frame "第二次水样测试中" {
                    n335 = global read "与总氮交互全局.vi" "总氮状态告警区"() -> (w221:T10)
                    n336 = Unbundle By Name(w221) -> ("工作状态"=w224:T6)
                    n337 = Equal?(x=w224, y=T6."空闲" ("工作状态")) -> (x = y?=w222:bool)
                    n338 = case shown="真" w222 {
                      tunnel: [w225 平行样测试流程."存储平行样测试数据"] -> w220
                      frame False {
                        n339 = flat-sequence {
                          tunnel: [平行样测试流程."第二次水样测试中"] -> w225
                          frame #0 {
                            n340 = Wait (ms)(milliseconds to wait=u32 1000 ("等待时间（毫秒）")) -> ()  [unwired: 1 out]
                          }
                          frame #1 {
                          }
                        }
                      }
                      frame True {
                        n341 = global read "与总氮交互全局.vi" "总氮测量数据区"() -> (w228:T11)
                        n342 = Unbundle By Name(w228) -> ("水样数据时间"=w231:timestamp, "水样实测值"=w232:sgl)
                        n343 = global read "平行样测试全局变量.vi" "总氮"() -> (w229:T12)
                        n344 = Bundle By Name(cluster=w229, "第二次水样测试时间"=w231, "第二次水样浓度值"=w232) -> (w230:T12)
                        n345 = global write "平行样测试全局变量.vi" "总氮"(w230) -> ()
                      }
                    }
                  }
                  frame "存储平行样测试数据" {
                    n346 = global read "平行样测试全局变量.vi" "总氮"() -> (w234:T12)
                    n347 = call "平行样测试数据写入.vi"("data"=w234) -> ()  [unwired: 10 in, 1 out]
                  }
                  frame "结束" {
                  }
                }
                n348 = feedback-in #15(w153) -> ()
              }
            }
            n349 = Compound Arithmetic op=AND ("复合运算")(w145, w141, w144, w140, w138) -> (w131:bool)
          }
        }
        n350 = case shown="假" w96 {
          tunnel: w114 -> [w117 w126]
          tunnel: [w116 w125] -> w112
          tunnel: w94 -> [w115 _]
          frame False {
            n351 = Select(t=enum16{"初始化", "采配水启动", "等待", "配水", "排水", "结束"}."结束" ("枚举"), s=w115, f=w117) -> (s? t:f=w116:enum16{"初始化", "采配水启动", "等待", "配水", "排水", "结束"})
          }
          frame True {
            n352 = global read "与采配水交互全局.vi" "状态"() -> (w124:T9)
            n353 = Unbundle By Name(w124) -> ("R0"=w123:i16)
            n354 = Equal To 0?(x=w123) -> (x = 0?=w120:bool)
            n355 = Greater?(x=w123, y=i16 6) -> (0:w121:bool)
            n356 = Or(x=w120, y=w121) -> (x .or. y?=w119:bool)
            n357 = Select(t=enum16{"初始化", "采配水启动", "等待", "配水", "排水", "结束"}."排水" ("枚举"), s=w119, f=w126) -> (s? t:f=w125:enum16{"初始化", "采配水启动", "等待", "配水", "排水", "结束"})
          }
        }
        n358 = Select(t=enum16{"初始化", "采配水启动", "等待", "配水", "排水", "结束"}."结束", s=w95, f=w112) -> (s? t:f=w111:enum16{"初始化", "采配水启动", "等待", "配水", "排水", "结束"})
      }
      frame "排水" {
        n359 = Increment(x=w591) -> (x+1=w587:enum16{"初始化", "采配水启动", "等待", "配水", "排水", "结束"})
        n360 = Enqueue Element At Opposite End(queue=w592, element=T2 {"命令"="单个写入", {"starting address"=303, "holding register value"=1}} ("元素")) -> ()  [unwired: 2 in, 3 out]
        n361 = Select(t=enum16{"初始化", "采配水启动", "等待", "配水", "排水", "结束"}."结束", s=w588, f=w587) -> (s? t:f=w586:enum16{"初始化", "采配水启动", "等待", "配水", "排水", "结束"})
      }
      frame "结束" {
        n362 = Increment(x=w598) -> (x+1=w597:enum16{"初始化", "采配水启动", "等待", "配水", "排水", "结束"})
        n363 = global write "质控测完标志全局 1.vi" "质控流程中"(FALSE ("质控流程中")) -> ()
      }
    }
    "枚举" <- w39
    n364 = Format Into String(format string="%s,当前运行时间%d秒" ("格式字符串"), w33, w32) -> ()  [unwired: 2 in, 2 out]
  }
  n365 = Cancel Notification(0:w15) -> (8:w14:refnum<notifier>)  [unwired: 1 in, 2 out]
  n366 = Release Notifier(notifier=w14) -> ()  [unwired: 2 in, 3 out]
